vi "Configure Sparse Marker [SM].vi"(5 "Destination Terminal (None)":string(combo) caption="destination terminal (None)", 6 "Indexes Array":i64[](array[numeric]) caption="indexes array", 7 "Number Indexes":i64 caption="number indexes" format="%.0g", 8 "error in (no error)":errorcluster, 9 "Waveform Handle":i32 caption="waveform handle" format="%.0g", 10 "Marker Name (\"\")":string caption="marker name (\"\")", 11 "CS++Fgen in":refnum<class "CS++Fgen.lvclass">) -> (0 "error out":errorcluster, 3 "CS++Fgen out":refnum<class "CS++Fgen.lvclass">)   [LabVIEW 2013, in "CS++Fgen.lvlib" / "CS++Fgen.lvclass"]
doc: "This VI configures the common sparse marker properties. These properties are the sparse marker waveform handle and destination.\n \nThis VI also configures which waveform and sample number the output is associated with.\n\nNote:\n\n(1) This VI is part of the IviFgenSparseMarker [SM] extension group."
uses:
  CS++Fgen.lvclass
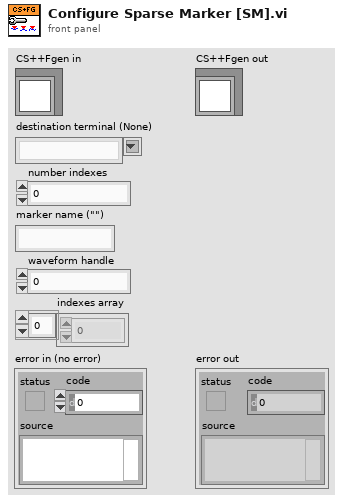
[diagram p1: front panel]
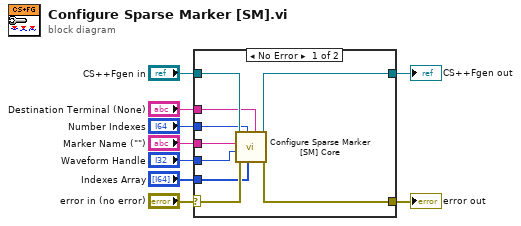
[diagram p0: block diagram]
diagram:
  n1 = case shown="No Error" "error in (no error)" {
    selector: "error in (no error)" -> [w16 w20]
    tunnel: [w15 w20] -> w8
    tunnel: [w17 w19] -> w6
    tunnel: "CS++Fgen in" -> [w18 w19]
    tunnel: "Marker Name (\"\")" -> [w14 _]
    tunnel: "Destination Terminal (None)" -> [w11 _]
    tunnel: "Number Indexes" -> [w12 _]
    tunnel: "Waveform Handle" -> [w13 _]
    tunnel: "Indexes Array" -> [w10 _]
    frame No Error {
      n2 = call-dynamic "Configure Sparse Marker [SM] Core.vi"("Destination Terminal (None)"=w11, "Indexes Array"=w10, "Number Indexes"=w12, "error in (no error)"=w16, "Waveform Handle"=w13, "Marker Name (\"\")"=w14, "CS++Fgen in"=w18) -> ("error out"=w15:errorcluster, "CS++Fgen out"=w17:refnum<class "CS++Fgen.lvclass">)  [unwired: 3 in]
    }
    frame Error {
    }
  }
  "error out" <- w8
  "CS++Fgen out" <- w6
